vi "Acquire.vi"(0 "Acq Settings in":T2 {"Config Settings"."Simulated Sensor Injection" scale=0.0..100.0}, 1 "Acquisition Context in":T1, 2 "Calibration in":refnum<k21>, 3 "UI":refnum<queue>, 4 "Data Notifier":refnum<notifier>, 5 "Queue A - Processing":refnum<queue>, 6 "Queue B -TDMS Raw":refnum<queue>, 7 "error in (no error)":errorcluster) -> (20 "Acq Settings out":T2 {"Config Settings"."Simulated Sensor Injection" scale=0.0..100.0}, 21 "Acquisition Context out":T1, 22 "Calibration out":refnum<k21>, 23 "Acknowledged?":bool, 27 "error out":errorcluster)   [LabVIEW 2026, in "Acquisition.lvlib"]
doc: "Perform the acquisition. Replace the contents of this diagram with calls to acquisition hardware."
uses:
  Acquisition.lvlib
  controls/UI/Acq Settings.ctl
  Instrument Specifications Configuration.ctl
  Instrument Specifications Cluster Configuration.ctl
  controls/UI/Measurement Role.ctl
  controls/UI/Config Settings.ctl
  Acquisition Context.ctl
  support/Architecture/Message Queue/Message Cluster.ctl
  <vilib>/DAQmx/read.llb/DAQmx Read (Analog 1D Wfm NChan NSamp).vi
  <vilib>/DAQmx/miscellaneous.llb/DAQmx Fill In Error Info.vi
  support/Architecture/Message Queue/Enqueue Message (Single).vi
  <vilib>/Analysis/NI_AALBase.lvlib
  support/Architecture/Message Queue/Message Queue.lvlib
  Settings/Settings.lvlib
  controls/UI/UUT Display Data.ctl
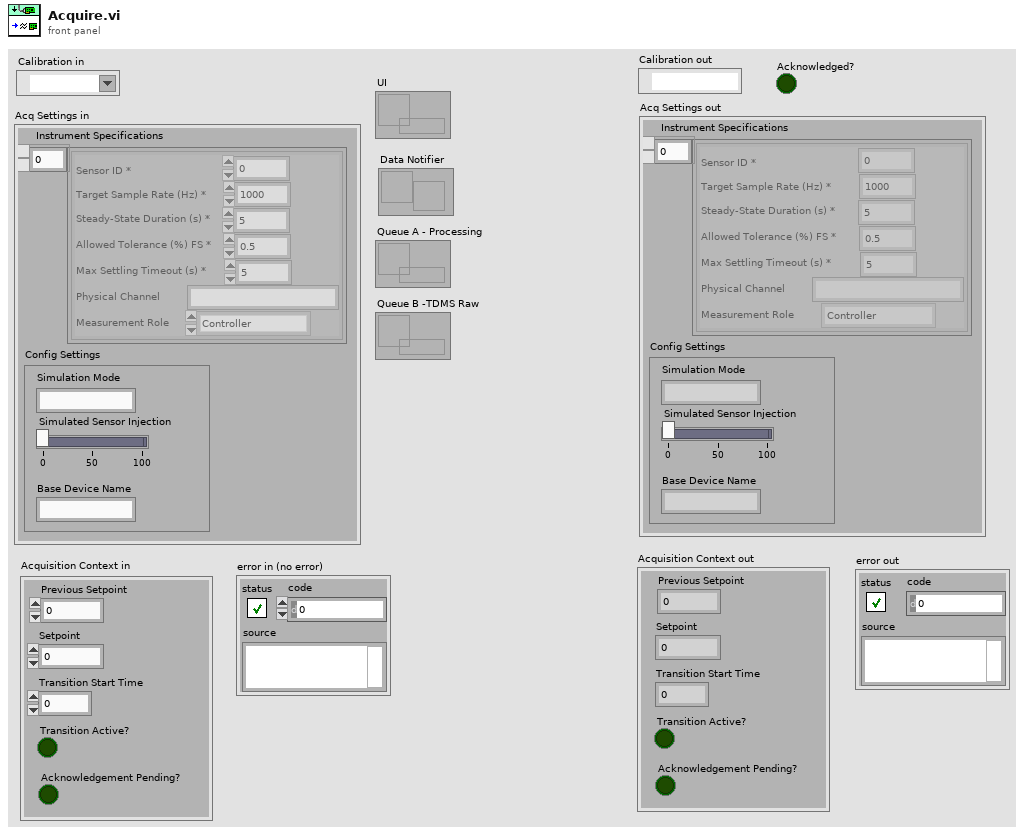
[diagram p1: front panel]
types:
  T1 = typedef "Acquisition.lvlib/Acquisition Context.ctl" = cluster{"Setpoint":dbl, "Previous Setpoint":dbl, "Transition Start Time":dbl, "Transition Active?":bool, "Acknowledgement Pending?":bool}
  T2 = typedef "Acq Settings.ctl" = cluster{"Instrument Specifications":T3, "Config Settings":T6}
  T3 = typedef "Acquisition.lvlib/Instrument Specifications Configuration.ctl" = T4[]
  T4 = typedef "Acquisition.lvlib/Instrument Specifications Cluster Configuration.ctl" = cluster{"Sensor ID *":i32, "Target Sample Rate (Hz) *":dbl, "Steady-State Duration (s) *":i32, "Allowed Tolerance (%) FS *":dbl, "Max Settling Timeout (s) *":i32, "Physical Channel":string, "Measurement Role":T5}
  T5 = typedef "Settings.lvlib/Measurement Role.ctl" = enum16{"Controller", "Reference", "UUT", "Disable", "All"}
  T6 = typedef "Config Settings.ctl" = cluster{"Simulated Sensor Injection":dbl, "Base Device Name":string, "Simulation Mode":string}
  T7 = typedef "UUT Display Data.ctl" = cluster{"Waveforms":waveform(dbl)[], "SensorIDs":i32[]}
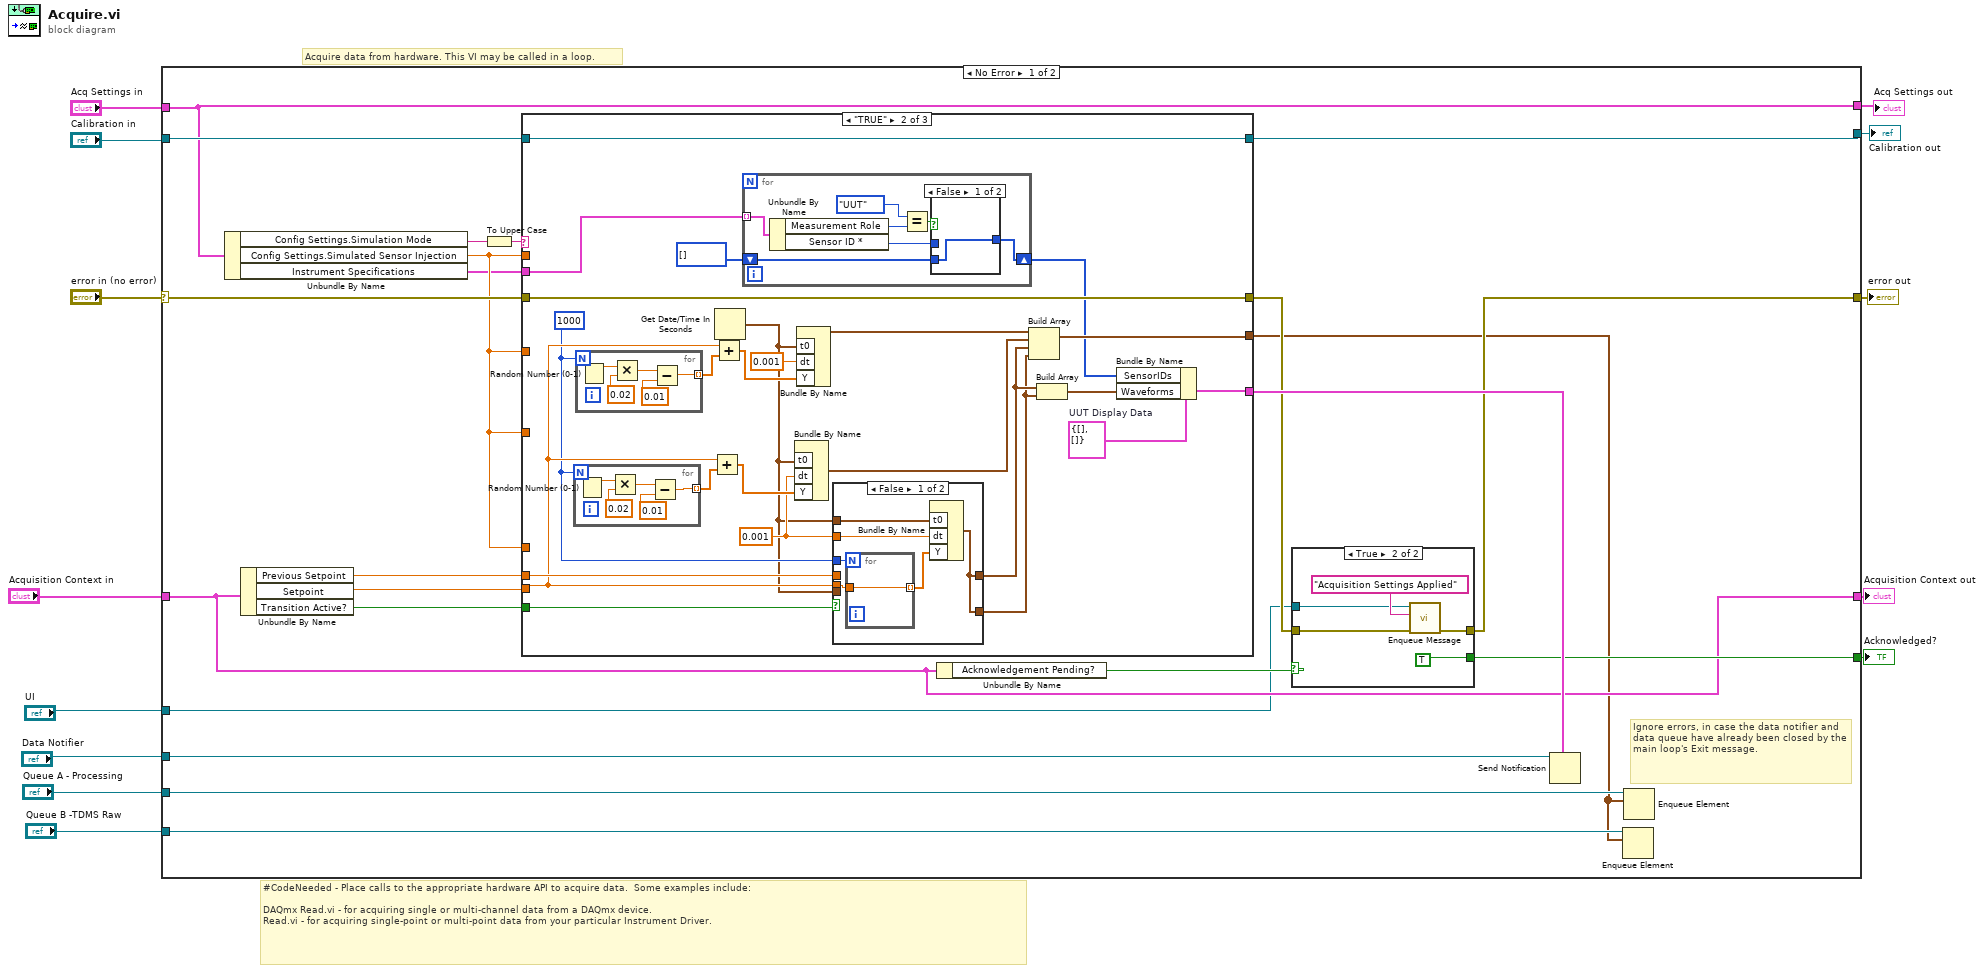
[diagram p0: block diagram]
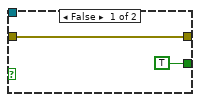
[diagram p2: hidden frame]
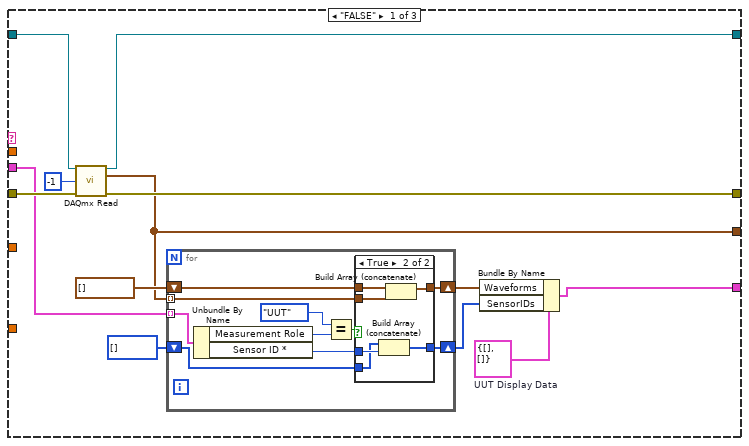
[diagram p3: hidden frame]
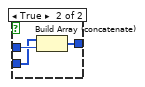
[diagram p5: hidden frame]
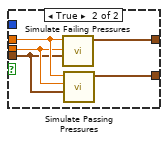
[diagram p6: hidden frame]
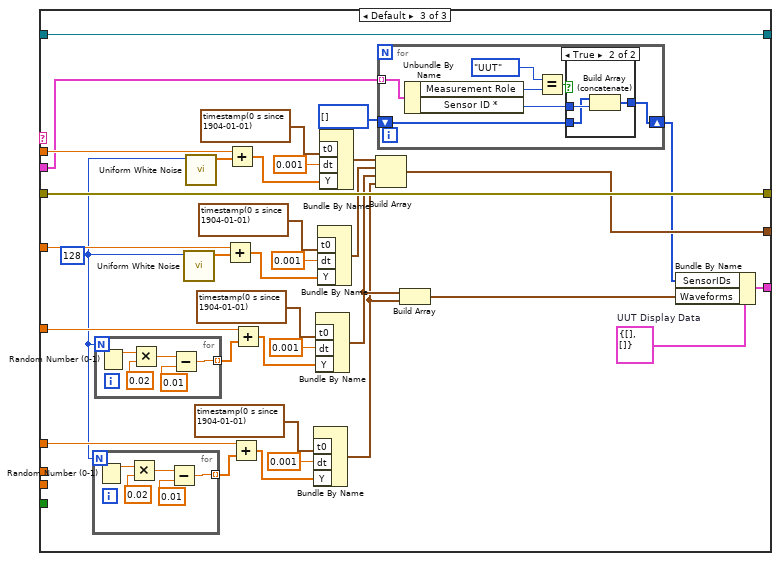
[diagram p7: hidden frame]
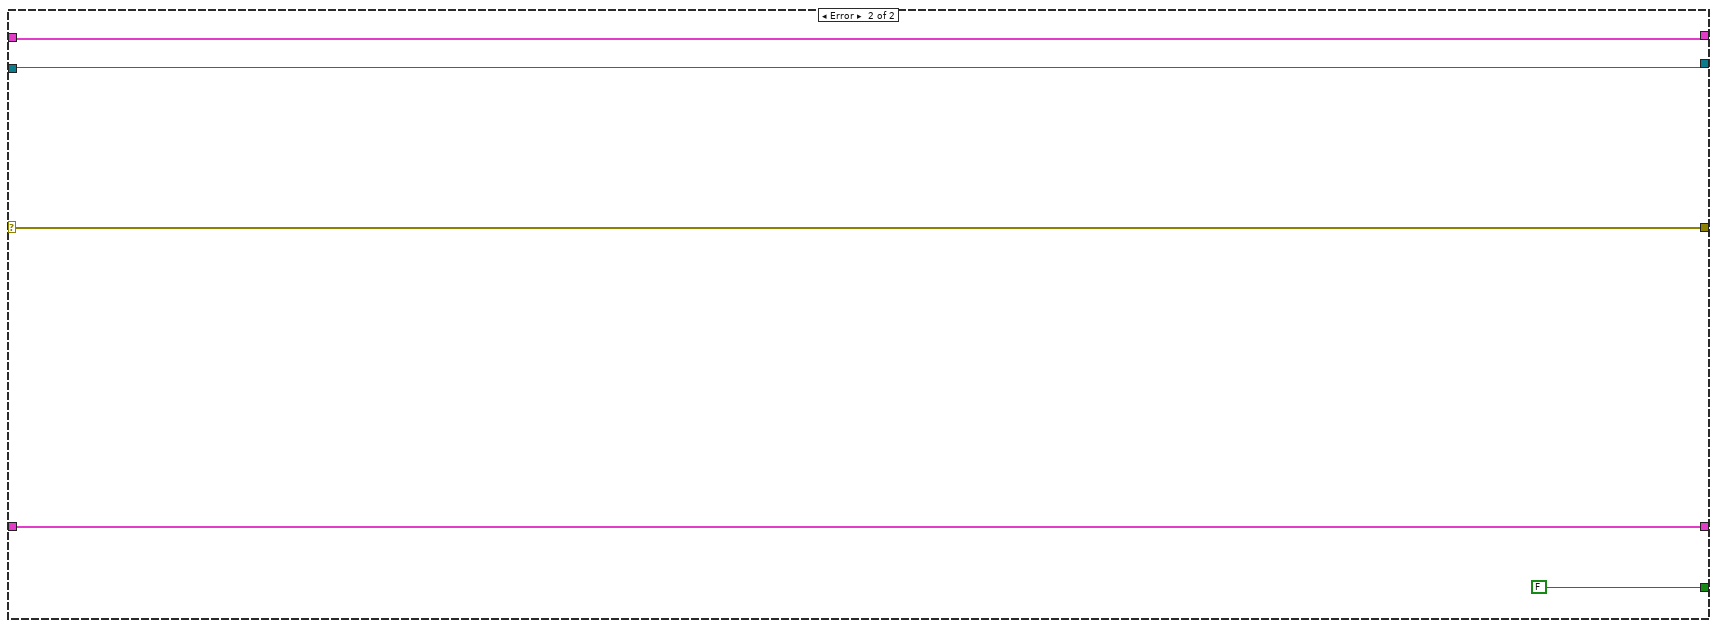
[diagram p9: hidden frame]
diagram:
  # "Acquire data from hardware. This VI may be called in a loop."
  # "#CodeNeeded - Place calls to the appropriate hardware API to acquire data.  Some examples include:\n\nDAQmx Read.vi - for acquiring single or multi-channel data from a DAQmx device.\nRead.vi - for acquiring single-point or multi-point data from your particular Instrument Driver."
  n1 = case shown="No Error" "error in (no error)" {
    selector: "error in (no error)" -> [w31 w188]
    tunnel: [w19 w188] -> w12
    tunnel: "Acq Settings in" -> [w28 w189]
    tunnel: [w28 w189] -> w6
    tunnel: "Data Notifier" -> [w35 _]
    tunnel: "Queue B -TDMS Raw" -> [w34 _]
    tunnel: "Calibration in" -> [w33 w187]
    tunnel: [w32 w187] -> w9
    tunnel: "Queue A - Processing" -> [w30 _]
    tunnel: "Acquisition Context in" -> [w17 w185]
    tunnel: [w18 FALSE] -> w4
    tunnel: [w17 w185] -> w3
    tunnel: "UI" -> [w16 _]
    frame No Error {
      # "Ignore errors, in case the data notifier and data queue have already been closed by the main loop's Exit message."
      n2 = Unbundle By Name(w28) -> ("Config Settings.Simulation Mode"=w27:string, "Config Settings.Simulated Sensor Injection"=w25:dbl, "Instrument Specifications"=w15:T3)
      n3 = Unbundle By Name(w17) -> ("Previous Setpoint"=w24:dbl, "Setpoint"=w23:dbl, "Transition Active?"=w22:bool)
      n4 = To Upper Case(1:w27) -> (0:w26:string)
      n5 = case shown="\"TRUE\"" w26 {
        tunnel: w33 -> [w55 w97 w163]
        tunnel: [w52 w97 w163] -> w32
        tunnel: w31 -> [w53 w89 w161]
        tunnel: [w51 w89 w161] -> w20
        tunnel: [w43 w74 w132] -> w29
        tunnel: w25 -> [_ _ w160]
        tunnel: w25 -> [_ _ w152]
        tunnel: w25 -> [_ _ w149]
        tunnel: w25 -> [_ _ w140]
        tunnel: w24 -> [_ w88 _]
        tunnel: w23 -> [_ w87 _]
        tunnel: w22 -> [_ w86 _]
        tunnel: w15 -> [w50 w79 w135]
        tunnel: [w48 w80 w136] -> w14
        frame "FALSE" {
          w46 = T7 {"Waveforms"=[], "SensorIDs"=[]}  # UUT Display Data
          n6 = call-poly <vilib>:"DAQmx Read.vi"("task/channels in"=w55, "number of samples per channel"=-1, "error in"=w53) -> ("task out"=w52:refnum<k21>, "data"=w48:waveform(dbl)[], "error out"=w51:errorcluster)  [unwired: 10 in]
          n7 = for {
            tunnel: w50 -> [w65] mode=indexing
            tunnel: w48 -> [w63] mode=indexing
            shift-right: [w62] -> w45
            shift-left: waveform(dbl)[] [] -> [w61]
            shift-right: [w57] -> w44
            shift-left: i32[] [] -> [w56]
            n8 = Unbundle By Name(w65) -> ("Measurement Role"=w59:T5, "Sensor ID *"=w58:i32)
            n9 = Equal?(x=Measurement_Role."UUT" ("Measurement Role"), y=w59) -> (x = y?=w64:bool)
            n10 = case shown="True" w64 {
              tunnel: w63 -> [_ w73]
              tunnel: [w67 w72] -> w62
              tunnel: w61 -> [w67 w71]
              tunnel: w58 -> [_ w70]
              tunnel: [w66 w69] -> w57
              tunnel: w56 -> [w66 w68]
              frame False {
              }
              frame True {
                n11 = Build Array (concatenate)(w68, w70) -> (w69:i32[])
                n12 = Build Array (concatenate)(w71, w73) -> (w72:waveform(dbl)[])
              }
            }
          }
          n13 = Bundle By Name(cluster=w46, "Waveforms"=w45, "SensorIDs"=w44) -> (w43:T7)
        }
        frame "TRUE" {
          w77 = T7 {"Waveforms"=[], "SensorIDs"=[]}  # UUT Display Data
          w85 = 1000
          w84 = 0.001 ("dt")
          n14 = for {
            N: w85 -> [_]
            tunnel: [w121] -> w92 mode=indexing
            n15 = Random Number (0-1)() -> (number: 0 to 1=w124:dbl)
            n16 = Multiply(x=w124, y=0.02) -> (x*y=w123:dbl)
            n17 = Subtract(x=w123, y=0.01) -> (x-y=w121:dbl)
          }
          n18 = for {
            N: w85 -> [_]
            tunnel: [w126] -> w94 mode=indexing
            n19 = Random Number (0-1)() -> (number: 0 to 1=w129:dbl)
            n20 = Multiply(x=w129, y=0.02) -> (x*y=w128:dbl)
            n21 = Subtract(x=w128, y=0.01) -> (x-y=w126:dbl)
          }
          n22 = Add(x=w87, y=w92) -> (x+y=w93:dbl[])
          n23 = Add(x=w87, y=w94) -> (x+y=w95:dbl[])
          n24 = Get Date/Time In Seconds() -> (seconds since 1Jan1904=w83:timestamp)
          n25 = for {
            tunnel: w79 -> [w104] mode=indexing
            shift-right: [w99] -> w76
            shift-left: i32[] [] -> [w98]
            n26 = Unbundle By Name(w104) -> ("Measurement Role"=w101:T5, "Sensor ID *"=w100:i32)
            n27 = Equal?(x=Measurement_Role."UUT" ("Measurement Role"), y=w101) -> (x = y?=w103:bool)
            n28 = case shown="False" w103 {
              tunnel: w100 -> [_ w108]
              tunnel: [w105 w107] -> w99
              tunnel: w98 -> [w105 w106]
              frame False {
              }
              frame True {
                n29 = Build Array (concatenate)(w106, w108) -> (w107:i32[])
              }
            }
          }
          n30 = Bundle By Name("t0"=w83, "dt"=w84, "Y"=w93) -> (w90:waveform(dbl))  [unwired: 1 in]
          n31 = Bundle By Name("t0"=w83, "dt"=0.001, "Y"=w95) -> (w91:waveform(dbl))  [unwired: 1 in]
          n32 = case shown="False" w86 {
            tunnel: [w109 w120] -> w82
            tunnel: [w109 w119] -> w81
            tunnel: w88 -> [_ w118]
            tunnel: w87 -> [w113 w117]
            tunnel: w85 -> [w114 _]
            tunnel: w84 -> [w111 _]
            tunnel: w83 -> [w110 _]
            tunnel: w83 -> [_ w116]
            frame False {
              n33 = for {
                N: w114 -> [_]
                tunnel: w113 -> [w115]
                tunnel: [w115] -> w112 mode=indexing
              }
              n34 = Bundle By Name("t0"=w110, "dt"=w111, "Y"=w112) -> (w109:waveform(dbl))  [unwired: 1 in]
            }
            frame True {
              n35 = call "Simulate Failing Pressures.vi"("seconds since 1Jan1904"=w116, "Pf"=w117, "Pi"=w118) -> ("Simulated Waveform"=w120:waveform(dbl))  [unwired: 7 in, 1 out]
              n36 = call "Simulate Passing Pressures.vi"("seconds since 1Jan1904"=w116, "Pf"=w117, "Pi"=w118) -> ("Simulated Waveform"=w119:waveform(dbl))  [unwired: 7 in, 1 out]
            }
          }
          n37 = Build Array(w91, w90, w82, w81) -> (w80:waveform(dbl)[])
          n38 = Build Array(w82, w81) -> (w75:waveform(dbl)[])
          n39 = Bundle By Name(cluster=w77, "SensorIDs"=w76, "Waveforms"=w75) -> (w74:T7)
        }
        frame Default {
          w132 = T7 {"Waveforms"=[], "SensorIDs"=[]}  # UUT Display Data
          w139 = 128 ("samples")
          n40 = for {
            N: w139 -> [_]
            tunnel: [w175] -> w141 mode=indexing
            n41 = Random Number (0-1)() -> (number: 0 to 1=w178:dbl)
            n42 = Multiply(x=w178, y=0.02) -> (x*y=w177:dbl)
            n43 = Subtract(x=w177, y=0.01) -> (x-y=w175:dbl)
          }
          n44 = for {
            N: w139 -> [_]
            tunnel: [w180] -> w147 mode=indexing
            n45 = Random Number (0-1)() -> (number: 0 to 1=w183:dbl)
            n46 = Multiply(x=w183, y=0.02) -> (x*y=w182:dbl)
            n47 = Subtract(x=w182, y=0.01) -> (x-y=w180:dbl)
          }
          n48 = call <vilib>:"Uniform White Noise.vi"("samples"=w139) -> ("uniform white noise"=w156:dbl[])  [unwired: 9 in, 1 out]
          n49 = call <vilib>:"Uniform White Noise.vi"("samples"=w139) -> ("uniform white noise"=w162:dbl[])  [unwired: 9 in, 1 out]
          n50 = Add(x=w152, y=w156) -> (x+y=w155:dbl[])
          n51 = Add(x=w160, y=w162) -> (x+y=w159:dbl[])
          n52 = Add(x=w140, y=w141) -> (x+y=w142:dbl[])
          n53 = Add(x=w149, y=w147) -> (x+y=w148:dbl[])
          n54 = Bundle By Name("t0"=timestamp(0 s since 1904-01-01), "dt"=0.001, "Y"=w142) -> (w137:waveform(dbl))  [unwired: 1 in]
          n55 = Bundle By Name("t0"=timestamp(0 s since 1904-01-01), "dt"=0.001, "Y"=w148) -> (w138:waveform(dbl))  [unwired: 1 in]
          n56 = Bundle By Name("t0"=timestamp(0 s since 1904-01-01), "dt"=0.001, "Y"=w155) -> (w146:waveform(dbl))  [unwired: 1 in]
          n57 = Bundle By Name("t0"=timestamp(0 s since 1904-01-01), "dt"=0.001, "Y"=w159) -> (w145:waveform(dbl))  [unwired: 1 in]
          n58 = Build Array(w145, w146, w138, w137) -> (w136:waveform(dbl)[])
          n59 = for {
            tunnel: w135 -> [w170] mode=indexing
            shift-right: [w165] -> w133
            shift-left: i32[] [] -> [w164]
            n60 = Unbundle By Name(w170) -> ("Measurement Role"=w167:T5, "Sensor ID *"=w166:i32)
            n61 = Equal?(x=Measurement_Role."UUT" ("Measurement Role"), y=w167) -> (x = y?=w169:bool)
            n62 = case shown="True" w169 {
              tunnel: w166 -> [_ w174]
              tunnel: [w171 w173] -> w165
              tunnel: w164 -> [w171 w172]
              frame False {
              }
              frame True {
                n63 = Build Array (concatenate)(w172, w174) -> (w173:i32[])
              }
            }
          }
          n64 = Build Array(w138, w137) -> (w134:waveform(dbl)[])
          n65 = Bundle By Name(cluster=w132, "SensorIDs"=w133, "Waveforms"=w134) -> ()  [unwired: 1 out]
        }
      }
      n66 = Unbundle By Name(w17) -> ("Acknowledgement Pending?"=w21:bool)
      n67 = case shown="True" w21 {
        tunnel: w20 -> [w37 w41]
        tunnel: [w37 w40] -> w19
        tunnel: [TRUE TRUE] -> w18
        tunnel: w16 -> [_ w38]
        frame False {
        }
        frame True {
          n68 = call-poly "Enqueue Message.vi"("error in (no error)"=w41, "Message"="Acquisition Settings Applied", "Message Queue"=w38) -> ("error out"=w40:errorcluster)  [unwired: 7 in, 1 out]
        }
      }
      n69 = Send Notification(notification=w29, notifier=w35) -> ()  [unwired: 1 in, 2 out]
      n70 = Enqueue Element(queue=w34, element=w14) -> ()  [unwired: 2 in, 3 out]
      n71 = Enqueue Element(queue=w30, element=w14) -> ()  [unwired: 2 in, 3 out]
    }
    frame Error {
    }
  }
  "error out" <- w12
  "Calibration out" <- w9
  "Acq Settings out" <- w6
  "Acknowledged?" <- w4
  "Acquisition Context out" <- w3
